vi "Reverse Sort Test.vi"(11 "Error In":errorcluster) -> (15 "Error Out":errorcluster)   [LabVIEW 2021, in "Test Files.lvlib"]
doc: "This VI has test cases for checking sorting array in reverse order."
uses:
  Test Files.lvlib
  <vilib>/addons/_JKI Toolkits/Caraya/classes/Test/Test.lvclass
  <vilib>/addons/_JKI Toolkits/Caraya/classes/Assert/Assert.lvclass
  CustomSortPath.lvlib
  <vilib>/addons/_JKI Toolkits/Caraya/classes/Assert/Assert Equal Value_Variant.vi
panel:
  # "Sort in reverse order test"
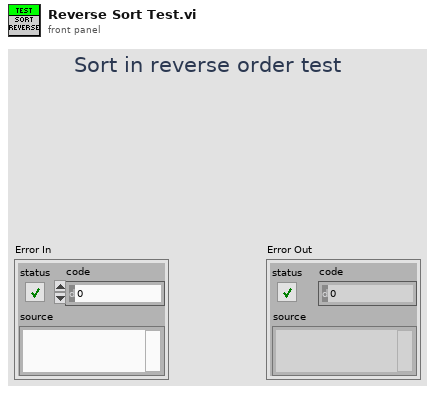
[diagram p1: front panel]
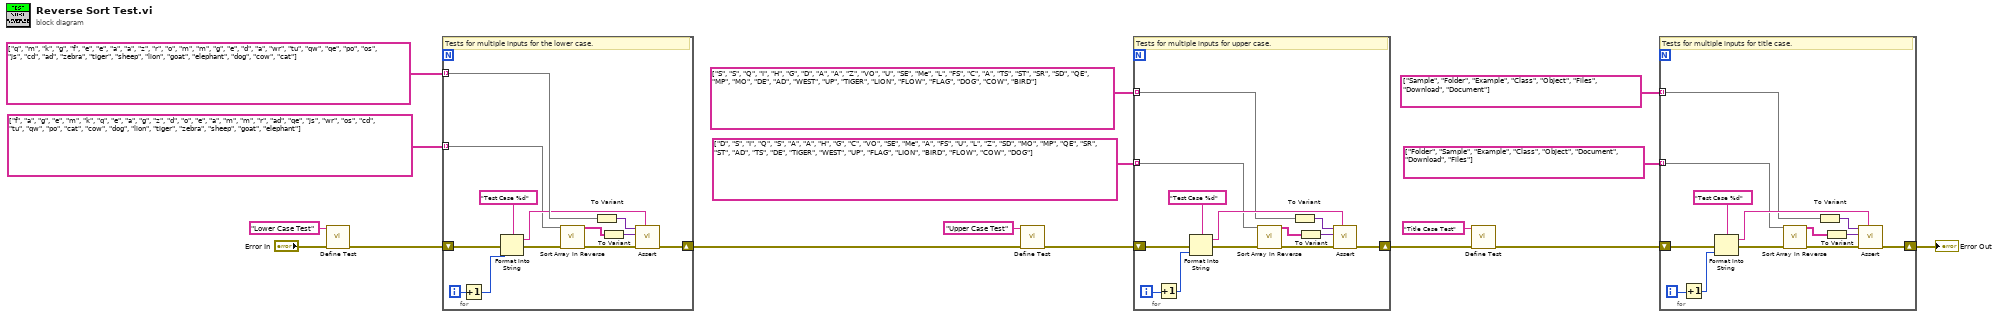
[diagram p0: block diagram]
diagram:
  n1 = call <vilib>:"Define Test.vi"("error in (no error)"="Error In", "Label (VI Title)"="Lower Case Test") -> ("error out"=w14:errorcluster)  [unwired: 8 in, 1 out]
  n2 = for {
    shift-right: [w29] -> w9
    shift-left: w14 -> [w28]
    tunnel: string[][] [["f", "a", "g", "e", "m", "k", "q", "e", "a"], ["g", "z", "d", "o", "e", "a", "m", "m", "r"], ["ad", "qe", "js", "wr", "os", "cd", "tu", "qw", "po"], ["cat", "cow", "dog", "lion", "tiger", "zebra", "sheep", "goat", "elephant"]] ("appended array") -> [w18] mode=indexing
    tunnel: string[][] [["q", "m", "k", "g", "f", "e", "e", "a", "a"], ["z", "r", "o", "m", "m", "g", "e", "d", "a"], ["wr", "tu", "qw", "qe", "po", "os", "js", "cd", "ad"], ["zebra", "tiger", "sheep", "lion", "goat", "elephant", "dog", "cow", "cat"]] ("appended array") -> [w22] mode=indexing
    i -> [w26]
    # "Tests for multiple inputs for the lower case."
    n3 = Increment(x=w26) -> (x+1=w17:i32)
    n4 = Format Into String(format string="Test Case %d", error in=w28, w17) -> (resulting string=w20:string, error out=w25:errorcluster)  [unwired: 1 in]
    n5 = call "Sort Array In Reverse.vi"("InputArray"=w18, "error in (no error)"=w25) -> ("SortedArray"=w19:string[], "error out"=w24:errorcluster)  [unwired: 12 in]
    n6 = To Variant(anything=w22) -> (Variant=w21:variant)
    n7 = To Variant(anything=w19) -> (Variant=w23:variant)
    n8 = call-poly <vilib>:"Assert.vi"("Label"=w20, "error in (no error)"=w24, "Y"=w23, "X"=w21) -> ("error out"=w29:errorcluster)  [unwired: 6 in, 1 out]
  }
  n9 = call <vilib>:"Define Test.vi"("error in (no error)"=w9, "Label (VI Title)"="Upper Case Test") -> ("error out"=w8:errorcluster)  [unwired: 8 in, 1 out]
  n10 = for {
    shift-right: [w42] -> w5
    shift-left: w8 -> [w41]
    tunnel: string[][] [["D", "S", "I", "Q", "S", "A", "A", "H", "G"], ["C", "VO", "SE", "Me", "A", "FS", "U", "L", "Z"], ["SD", "MO", "MP", "QE", "SR", "ST", "AD", "TS", "DE"], ["TIGER", "WEST", "UP", "FLAG", "LION", "BIRD", "FLOW", "COW", "DOG"]] ("appended array") -> [w33] mode=indexing
    tunnel: string[][] [["S", "S", "Q", "I", "H", "G", "D", "A", "A"], ["Z", "VO", "U", "SE", "Me", "L", "FS", "C", "A"], ["TS", "ST", "SR", "SD", "QE", "MP", "MO", "DE", "AD"], ["WEST", "UP", "TIGER", "LION", "FLOW", "FLAG", "DOG", "COW", "BIRD"]] ("appended array") -> [w32] mode=indexing
    i -> [w39]
    # "Tests for multiple inputs for upper case."
    n11 = Increment(x=w39) -> (x+1=w30:i32)
    n12 = Format Into String(format string="Test Case %d", error in=w41, w30) -> (resulting string=w34:string, error out=w38:errorcluster)  [unwired: 1 in]
    n13 = call "Sort Array In Reverse.vi"("InputArray"=w33, "error in (no error)"=w38) -> ("SortedArray"=w31:string[], "error out"=w37:errorcluster)  [unwired: 12 in]
    n14 = To Variant(anything=w32) -> (Variant=w35:variant)
    n15 = To Variant(anything=w31) -> (Variant=w36:variant)
    n16 = call-poly <vilib>:"Assert.vi"("Label"=w34, "error in (no error)"=w37, "Y"=w36, "X"=w35) -> ("error out"=w42:errorcluster)  [unwired: 6 in, 1 out]
  }
  n17 = call <vilib>:"Define Test.vi"("error in (no error)"=w5, "Label (VI Title)"="Title Case Test") -> ("error out"=w4:errorcluster)  [unwired: 8 in, 1 out]
  n18 = for {
    shift-right: [w55] -> w1
    shift-left: w4 -> [w54]
    tunnel: string[][] [["Folder", "Sample", "Example", "Class"], ["Object", "Document", "Download", "Files"]] ("appended array") -> [w46] mode=indexing
    tunnel: string[][] [["Sample", "Folder", "Example", "Class"], ["Object", "Files", "Download", "Document"]] ("appended array") -> [w45] mode=indexing
    i -> [w52]
    # "Tests for multiple inputs for title case."
    n19 = Increment(x=w52) -> (x+1=w43:i32)
    n20 = Format Into String(format string="Test Case %d", error in=w54, w43) -> (resulting string=w47:string, error out=w51:errorcluster)  [unwired: 1 in]
    n21 = call "Sort Array In Reverse.vi"("InputArray"=w46, "error in (no error)"=w51) -> ("SortedArray"=w44:string[], "error out"=w50:errorcluster)  [unwired: 12 in]
    n22 = To Variant(anything=w45) -> (Variant=w48:variant)
    n23 = To Variant(anything=w44) -> (Variant=w49:variant)
    n24 = call-poly <vilib>:"Assert.vi"("Label"=w47, "error in (no error)"=w50, "Y"=w49, "X"=w48) -> ("error out"=w55:errorcluster)  [unwired: 6 in, 1 out]
  }
  "Error Out" <- w1
